vi "DPT Gas Dry Encoder Input.vi"(0 "Number of Samples":i32=50, 2 "task/channels in":refnum<k21>="PortRead", 5 "Data Sample Period(mS)":u32=10, 11 "error in (no error)":errorcluster, 12 "ft3 Per Rotation":dbl format="%_3g", 13 "Ticks Per Rotation":dbl=400.0) -> (4 "ft3":dbl, 6 "dT":dbl, 8 "ft3 per Hour":dbl, 15 "error out":errorcluster)   [LabVIEW 2016]
uses:
  <vilib>/DAQmx/read.llb/DAQmx Read (Digital U8 1Chan 1Samp).vi
  <vilib>/DAQmx/miscellaneous.llb/DAQmx Fill In Error Info.vi
panel:
  out "Threes":i16
  out "Twos":i16
  out "Ones":i16
  out "Time, Encoder, Tick":dbl[][](array[numeric])
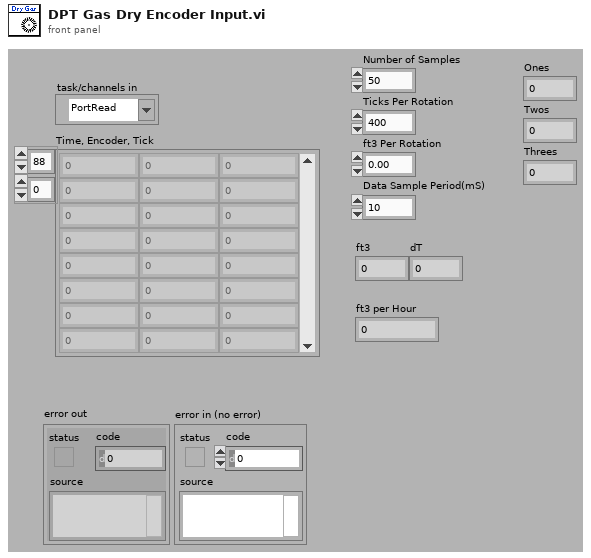
[diagram p1: front panel]
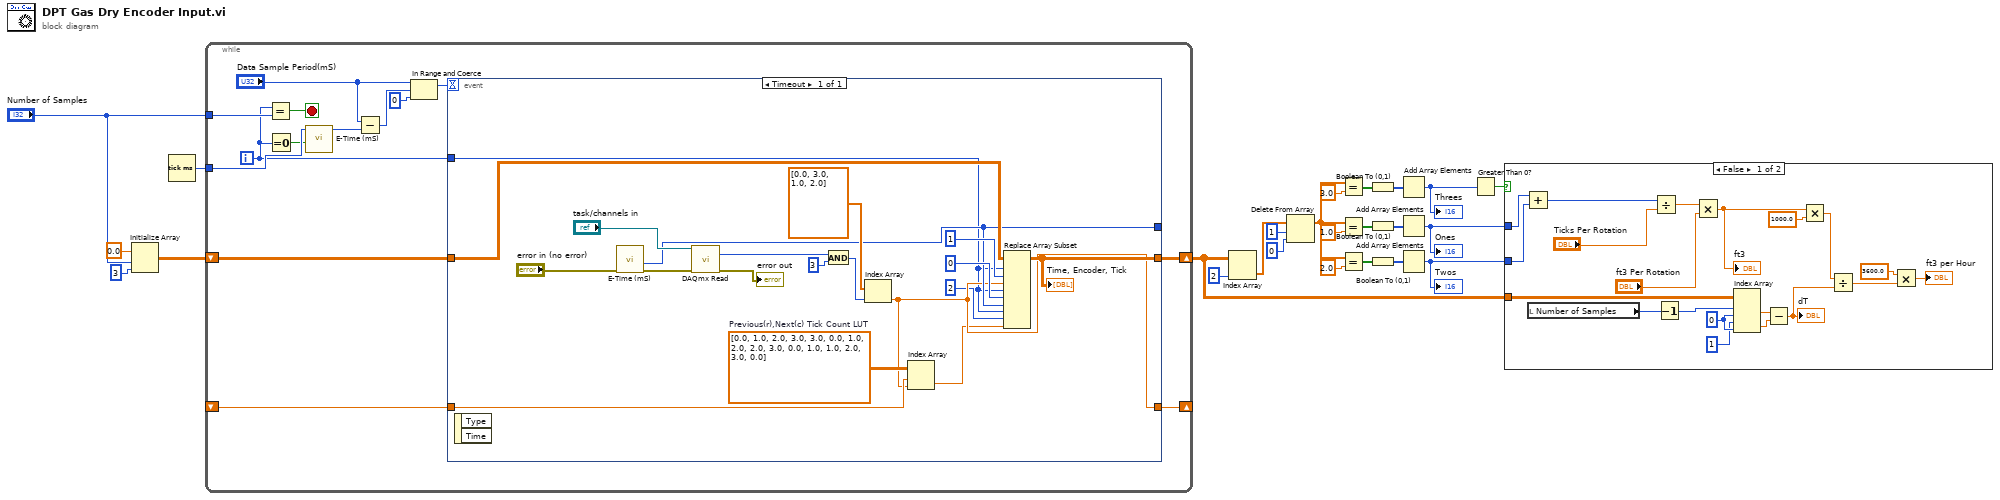
[diagram p0: block diagram]
diagram:
  n1 = Initialize Array(0.0 ("element"), "Number of Samples", 3 ("dimension size")) -> (w21:dbl[][])
  n2 = Tick Count (ms)() -> (millisecond timer value=w20:u32)
  n3 = while {
    tunnel: "Number of Samples" -> [w37]
    shift-right: [w35] -> w1
    shift-left: w21 -> [w36]
    tunnel: w20 -> [w29]
    shift-right: [w26] -> _
    shift-left: _ -> [w25]
    i -> [w27]
    stop <- w38 stop-if-true
    n4 = Equal?(x=w27, y=w37) -> (x = y?=w38:bool)
    n5 = Equal To 0?(x=w27) -> (x = 0?=w28:bool)
    n6 = call "E-Time (mS).vi"("Enter Start Time(mS)"=w29, "Reset"=w28) -> ("Time Since Last Run(mS)"=w32:u32)  [unwired: 7 in, 2 out]
    n7 = Subtract(x="Data Sample Period(mS)", y=w32) -> (x-y=w34:u32)
    n8 = In Range and Coerce(upper limit="Data Sample Period(mS)", x=w34, lower limit=u32 0) -> (coerced(x)=w30:u32)  [unwired: 1 out]
    n9 = event shown="[0] Timeout" {
      selector: _ -> [_]
      dyn-events: _ -> [_]
      timeout: w30 -> [_]
      tunnel: [w46] -> _
      tunnel: w36 -> [w54]
      tunnel: w27 -> [w41]
      tunnel: [w49] -> w35
      tunnel: [w44] -> w26
      tunnel: w25 -> [w45]
      event Timeout {
        w47 = dbl[][] [[0.0, 1.0, 2.0, 3.0], [3.0, 0.0, 1.0, 2.0], [2.0, 3.0, 0.0, 1.0], [1.0, 2.0, 3.0, 0.0]]  # Previous(r),Next(c) Tick Count LUT
        n10 = event-data() -> ()  [unwired: 1 in, 2 out]
        n11 = call "E-Time (mS).vi"("error in (no error)"="error in (no error)") -> ("error out"=w48:errorcluster, "Elapsed Time (mS)"=w46:u32)  [unwired: 8 in, 1 out]
        n12 = call-poly <vilib>:"DAQmx Read.vi"("task/channels in"="task/channels in", "error in"=w48) -> ("data"=w56:u8, "error out"=→"error out":errorcluster)  [unwired: 11 in, 1 out]
        n13 = And(x=w56, y=u8 3) -> (x .and. y?=w53:u8)
        n14 = Index Array(array=dbl[] [0.0, 3.0, 1.0, 2.0], index=w53) -> (element=w44:dbl)
        n15 = Index Array(array=w47, index (row)=w45, index (col)=w44) -> (element=w43:dbl)
        n16 = Replace Array Subset(array=w54, new element #1=w44, index (row) #1=w41, index (col) #1=1 ("disabled index (col)"), new element #2=w46, index (row) #2=w41, index (col) #2=0 ("disabled index (col)"), new element #3=w43, index (row) #3=w41, index (col) #3=2 ("index (row)")) -> (w49:dbl[][])
        "Time, Encoder, Tick" <- w49
      }
    }
  }
  n17 = Index Array(array=w1, index (col)=2 ("disabled index (col)")) -> (element=w2:dbl[])  [unwired: 1 in]
  n18 = Delete From Array(array=w2, length=1, index=0) -> (array with subset deleted=w9:dbl[])  [unwired: 1 out]
  n19 = Equal?(x=w9, y=3.0) -> (x = y?=w12:bool[])
  n20 = Equal?(x=w9, y=1.0) -> (x = y?=w17:bool[])
  n21 = Equal?(x=w9, y=2.0) -> (x = y?=w10:bool[])
  n22 = Boolean To (0,1)(Boolean=w12) -> (0, 1=w11:i16[])
  n23 = Boolean To (0,1)(Boolean=w17) -> (0, 1=w16:i16[])
  n24 = Boolean To (0,1)(Boolean=w10) -> (0, 1=w15:i16[])
  n25 = Add Array Elements(numeric array=w11) -> (sum=w5:i16)
  "Threes" <- w5
  n26 = Add Array Elements(numeric array=w16) -> (sum=w3:i16)
  "Ones" <- w3
  n27 = Add Array Elements(numeric array=w15) -> (sum=w4:i16)
  "Twos" <- w4
  n28 = Greater Than 0?(x=w5) -> (x > 0?=w6:bool)
  n29 = case shown="False" w6 {
    tunnel: w4 -> [w77 _]
    tunnel: w3 -> [w76 _]
    tunnel: w1 -> [w75 _]
    frame False {
      w65 = 0 ("disabled index (row)")
      n30 = Add(x=w76, y=w77) -> (x+y=w71:i16)
      n31 = local read "Number of Samples"() -> (w59:i32)
      n32 = Divide(x=w71, y="Ticks Per Rotation") -> (x/y=w69:dbl)
      n33 = Decrement(x=w59) -> (x-1=w58:i32)
      n34 = Multiply(x=w69, y="ft3 Per Rotation") -> (x*y=w63:dbl)
      "ft3" <- w63
      n35 = Index Array(array=w75, index (row) #1=w58, index (col) #1=w65, index (row) #2=1 ("disabled index (col)"), index (col) #2=w65) -> (element #1=w73:dbl, element #2=w74:dbl)
      n36 = Subtract(x=w73, y=w74) -> (x-y=w60:dbl)
      "dT" <- w60
      n37 = Multiply(x=w63, y=1000.0) -> (x*y=w61:dbl)
      n38 = Divide(x=w61, y=w60) -> (x/y=w68:dbl)
      n39 = Multiply(x=3600.0, y=w68) -> (x*y=→"ft3 per Hour":dbl)
    }
    frame True {
      # "Too Fast to Read Accurately"
    }
  }
